vi "PRBS64 Parallel Rx - N Lanes.vi"(7 "reset":bool, 9 "input valid":bool=TRUE, 11 "rx prbs":u64[](array[numeric])) -> (1 "output valid":bool, 3 "pattern mismatch":bool)   [LabVIEW 2023, in "Aurora64b66b Utilities FPGA.lvlib"]
uses:
  Aurora64b66b Utilities FPGA.lvlib
  Program Files/NI/LVAddons/niidl/1/instr.lib/_niInstr/Basic Elements/v1/FPGA/niInstr Basic Elements v1 FPGA.lvlib
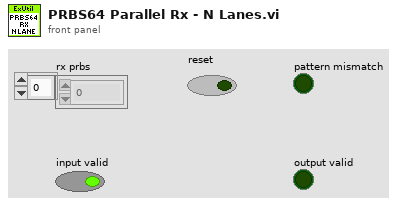
[diagram p1: front panel]
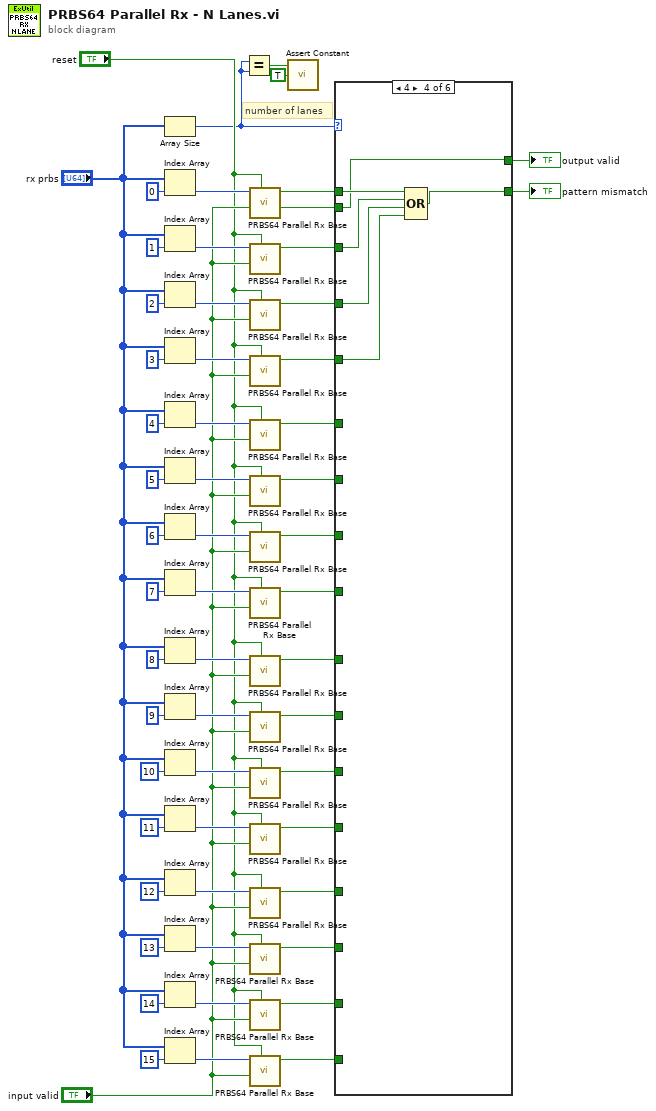
[diagram p0: block diagram]
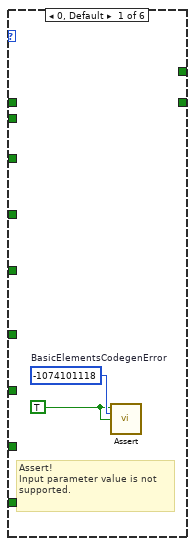
[diagram p2: hidden frame]
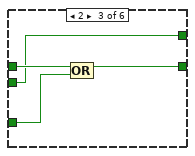
[diagram p4: hidden frame]
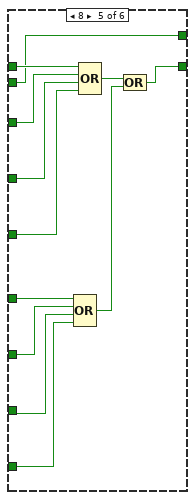
[diagram p5: hidden frame]
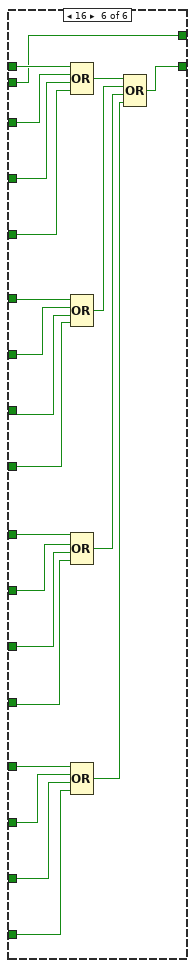
[diagram p6: hidden frame]
diagram:
  # "number of lanes"
  n1 = Array Size(array="rx prbs") -> (size(s)=w3:i32)
  n2 = Index Array(array="rx prbs", index=0) -> (element=w56:u64)
  n3 = Index Array(array="rx prbs", index=1) -> (element=w52:u64)
  n4 = Index Array(array="rx prbs", index=2) -> (element=w51:u64)
  n5 = Index Array(array="rx prbs", index=3) -> (element=w50:u64)
  n6 = Index Array(array="rx prbs", index=4) -> (element=w40:u64)
  n7 = Index Array(array="rx prbs", index=5) -> (element=w44:u64)
  n8 = Index Array(array="rx prbs", index=6) -> (element=w45:u64)
  n9 = Index Array(array="rx prbs", index=7) -> (element=w46:u64)
  n10 = Index Array(array="rx prbs", index=8) -> (element=w33:u64)
  n11 = Index Array(array="rx prbs", index=9) -> (element=w29:u64)
  n12 = Index Array(array="rx prbs", index=10) -> (element=w28:u64)
  n13 = Index Array(array="rx prbs", index=11) -> (element=w27:u64)
  n14 = Index Array(array="rx prbs", index=12) -> (element=w20:u64)
  n15 = Index Array(array="rx prbs", index=13) -> (element=w24:u64)
  n16 = Index Array(array="rx prbs", index=14) -> (element=w25:u64)
  n17 = Index Array(array="rx prbs", index=15) -> (element=w26:u64)
  n18 = Equal?(x=w3, y=w3) -> (x = y?=w2:bool)
  n19 = call "PRBS64 Parallel Rx Base.vi"("reset"="reset", "input valid"="input valid", "prbs rx"=w56) -> ("output valid"=w6:bool, "pattern mismatch"=w9:bool)  [unwired: 7 in]
  n20 = call "PRBS64 Parallel Rx Base.vi"("reset"="reset", "input valid"="input valid", "prbs rx"=w52) -> ("pattern mismatch"=w49:bool)  [unwired: 7 in, 1 out]
  n21 = call "PRBS64 Parallel Rx Base.vi"("reset"="reset", "input valid"="input valid", "prbs rx"=w51) -> ("pattern mismatch"=w48:bool)  [unwired: 7 in, 1 out]
  n22 = call "PRBS64 Parallel Rx Base.vi"("reset"="reset", "input valid"="input valid", "prbs rx"=w50) -> ("pattern mismatch"=w47:bool)  [unwired: 7 in, 1 out]
  n23 = call "PRBS64 Parallel Rx Base.vi"("reset"="reset", "input valid"="input valid", "prbs rx"=w40) -> ("pattern mismatch"=w38:bool)  [unwired: 7 in, 1 out]
  n24 = call "PRBS64 Parallel Rx Base.vi"("reset"="reset", "input valid"="input valid", "prbs rx"=w44) -> ("pattern mismatch"=w37:bool)  [unwired: 7 in, 1 out]
  n25 = call "PRBS64 Parallel Rx Base.vi"("reset"="reset", "input valid"="input valid", "prbs rx"=w45) -> ("pattern mismatch"=w36:bool)  [unwired: 7 in, 1 out]
  n26 = call "PRBS64 Parallel Rx Base.vi"("reset"="reset", "input valid"="input valid", "prbs rx"=w46) -> ("pattern mismatch"=w35:bool)  [unwired: 7 in, 1 out]
  n27 = call "PRBS64 Parallel Rx Base.vi"("reset"="reset", "input valid"="input valid", "prbs rx"=w33) -> ("pattern mismatch"=w18:bool)  [unwired: 7 in, 1 out]
  n28 = call "PRBS64 Parallel Rx Base.vi"("reset"="reset", "input valid"="input valid", "prbs rx"=w29) -> ("pattern mismatch"=w17:bool)  [unwired: 7 in, 1 out]
  n29 = call "PRBS64 Parallel Rx Base.vi"("reset"="reset", "input valid"="input valid", "prbs rx"=w28) -> ("pattern mismatch"=w16:bool)  [unwired: 7 in, 1 out]
  n30 = call "PRBS64 Parallel Rx Base.vi"("reset"="reset", "input valid"="input valid", "prbs rx"=w27) -> ("pattern mismatch"=w15:bool)  [unwired: 7 in, 1 out]
  n31 = call "PRBS64 Parallel Rx Base.vi"("reset"="reset", "input valid"="input valid", "prbs rx"=w20) -> ("pattern mismatch"=w14:bool)  [unwired: 7 in, 1 out]
  n32 = call "PRBS64 Parallel Rx Base.vi"("reset"="reset", "input valid"="input valid", "prbs rx"=w24) -> ("pattern mismatch"=w13:bool)  [unwired: 7 in, 1 out]
  n33 = call "PRBS64 Parallel Rx Base.vi"("reset"="reset", "input valid"="input valid", "prbs rx"=w25) -> ("pattern mismatch"=w12:bool)  [unwired: 7 in, 1 out]
  n34 = call "PRBS64 Parallel Rx Base.vi"("reset"="reset", "input valid"="input valid", "prbs rx"=w26) -> ("pattern mismatch"=w11:bool)  [unwired: 7 in, 1 out]
  n35 = call "Assert Constant.vi"("constant terminal"=w2, "enable show error"=TRUE) -> ()  [unwired: 14 in]
  n36 = case shown="4" w3 {
    tunnel: w9 -> [_ w61 w65 w71 w83 w105]
    tunnel: w49 -> [_ _ w64 w70 w81 w103]
    tunnel: w48 -> [_ _ _ w69 w77 w99]
    tunnel: w47 -> [_ _ _ w68 w76 w98]
    tunnel: w38 -> [_ _ _ _ w80 w102]
    tunnel: w37 -> [_ _ _ _ w79 w101]
    tunnel: w36 -> [_ _ _ _ w75 w97]
    tunnel: w35 -> [_ _ _ _ w74 w96]
    tunnel: w18 -> [_ _ _ _ _ w94]
    tunnel: w17 -> [_ _ _ _ _ w93]
    tunnel: w16 -> [_ _ _ _ _ w92]
    tunnel: w15 -> [_ _ _ _ _ w91]
    tunnel: w14 -> [_ _ _ _ _ w90]
    tunnel: w13 -> [_ _ _ _ _ w89]
    tunnel: w12 -> [_ _ _ _ _ w88]
    tunnel: w11 -> [_ _ _ _ _ w87]
    tunnel: [_ w61 w63 w67 w73 w95] -> w7
    tunnel: w6 -> [_ w60 w62 w66 w72 w84]
    tunnel: [_ w60 w62 w66 w72 w84] -> w5
    frame 0, Default {
      w59 = -1074101118  # BasicElementsCodegenError
      w58 = TRUE ("assert")
      # "Assert!\nInput parameter value is not supported."
      n37 = call "Assert.vi"("assert"=w58, "error code"=w59, "enable show error"=w58) -> ()  [unwired: 13 in]
    }
    frame 1 {
    }
    frame 2 {
      n38 = Compound Arithmetic op=OR(w65, w64) -> (w63:bool)
    }
    frame 4 {
      n39 = Compound Arithmetic op=OR(w71, w70, w69, w68) -> (w67:bool)
    }
    frame 8 {
      n40 = Compound Arithmetic op=OR(w80, w79, w75, w74) -> (w78:bool)
      n41 = Compound Arithmetic op=OR(w83, w81, w77, w76) -> (w82:bool)
      n42 = Compound Arithmetic op=OR(w82, w78) -> (w73:bool)
    }
    frame 16 {
      n43 = Compound Arithmetic op=OR(w105, w103, w99, w98) -> (w104:bool)
      n44 = Compound Arithmetic op=OR(w102, w101, w97, w96) -> (w100:bool)
      n45 = Compound Arithmetic op=OR(w94, w93, w92, w91) -> (w86:bool)
      n46 = Compound Arithmetic op=OR(w90, w89, w88, w87) -> (w85:bool)
      n47 = Compound Arithmetic op=OR(w104, w100, w86, w85) -> (w95:bool)
    }
  }
  "pattern mismatch" <- w7
  "output valid" <- w5
